vi "Problem1.7.vi"() -> ()   [LabVIEW 2018]
panel:
  out "output cluster":cluster{"First Name":string, "Last Name":string}
  in  "Input Cluster":cluster{"First Name":string, "Last Name":string}
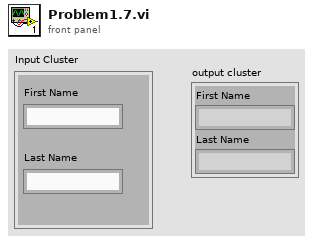
[diagram p1: front panel]
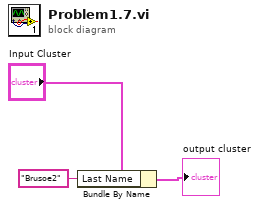
[diagram p0: block diagram]
diagram:
  n1 = Bundle By Name(cluster="Input Cluster", "Last Name"="Brusoe2") -> (→"output cluster":cluster{"First Name":string, "Last Name":string})
